vi "primer_2021_x64.vi"() -> ()   [LabVIEW 2021]
panel:
  out "PI":sgl format="%#.6g"
  in  "Operation":u8(ring) items=["sum", "subtract", "multiply", "divide", "square"]
  in  "Path to DLL":path=path "C:/Users/fl1ckje/Desktop/MathLib_x64.dll"
  out "z":i32=8
  in  "y":i32=2
  in  "x":i32=6
  # "Путь к DLL файлу библиотеки"
  # "Пример 1"
  # "Операция (функция) из DLL"
  # "Пример 2"
  # "Вызываем функцию float get_pi(), которая возвращает константу"
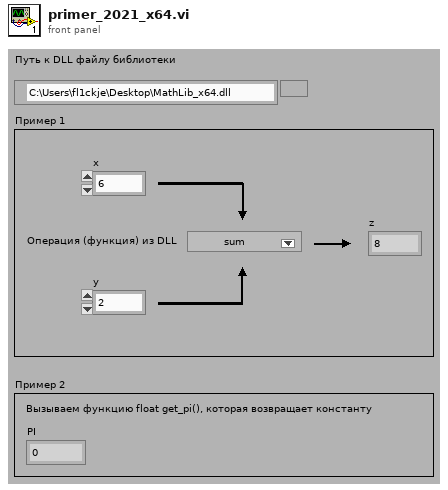
[diagram p1: front panel]
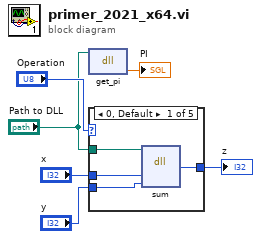
[diagram p0: block diagram]
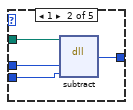
[diagram p2: hidden frame]
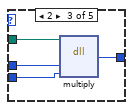
[diagram p3: hidden frame]
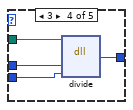
[diagram p4: hidden frame]
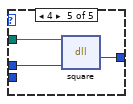
[diagram p5: hidden frame]
diagram:
  n1 = dll-call lib="C:/Users/fl1ckje/Desktop/MathLib_x64.dll" fn="get_pi"(path in="Path to DLL") -> ("return type"=→"PI":sgl)  [unwired: 2 in, 2 out]
  n2 = case shown="0, Default" "Operation" {
    tunnel: "Path to DLL" -> [w10 w11 w18 w20 w25]
    tunnel: "x" -> [w9 w14 w17 w22 w24]
    tunnel: "y" -> [w8 w13 w16 w21 _]
    tunnel: [w7 w12 w15 w19 w23] -> w3
    frame 0, Default {
      n3 = dll-call lib="C:/Users/fl1ckje/Desktop/MathLib_x64.dll" fn="sum"(path in=w10, "x"=w9, "y"=w8) -> ("return type"=w7:i32)  [unwired: 4 in, 2 out]
    }
    frame 1 {
      n4 = dll-call lib="C:/Users/fl1ckje/Desktop/MathLib_x86.dll" fn="subtract"(path in=w11, "x"=w14, "y"=w13) -> ("return type"=w12:i32)  [unwired: 4 in, 2 out]
    }
    frame 2 {
      n5 = dll-call lib="C:/Users/fl1ckje/Desktop/MathLib_x86.dll" fn="multiply"(path in=w18, "x"=w17, "y"=w16) -> ("return type"=w15:i32)  [unwired: 4 in, 2 out]
    }
    frame 3 {
      n6 = dll-call lib="C:/Users/fl1ckje/Desktop/MathLib_x86.dll" fn="divide"(path in=w20, "x"=w22, "y"=w21) -> ("return type"=w19:i32)  [unwired: 4 in, 2 out]
    }
    frame 4 {
      n7 = dll-call lib="C:/Users/fl1ckje/Desktop/MathLib_x86.dll" fn="square"(path in=w25, "x"=w24) -> ("return type"=w23:i32)  [unwired: 3 in, 2 out]
    }
  }
  "z" <- w3
